vi "filter_active_tracks_for_mature_tracks.vi"(1 "All Active Tracks":T1[](array[typedef])) -> (0 "All Mature Tracks":T1[](array[typedef]))   [LabVIEW 2019]
uses:
  WormTrackCluster.ctl
  StimulusObject.lvclass
  TrackTerminationReasonEnum.ctl
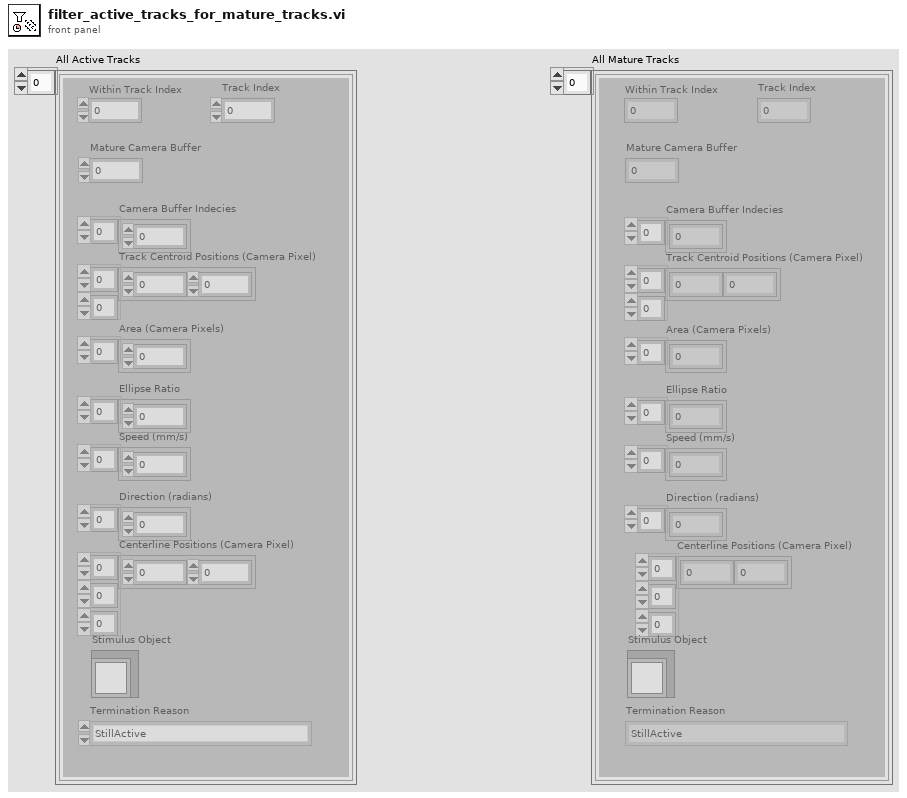
[diagram p1: front panel]
types:
  T1 = typedef "WormTrackCluster.ctl" = cluster{"Track Centroid Positions (Camera Pixel)":sgl[][], "Within Track Index":i32, "Camera Buffer Indecies":i32[], "Area (Camera Pixels)":i32[], "Speed (mm/s)":sgl[], "Direction (radians)":sgl[], "Centerline Positions (Camera Pixel)":sgl[][][], "Ellipse Ratio":sgl[], "Stimulus Object":refnum<class "StimulusObject.lvclass">, "Termination Reason":T2, "Track Index":i32, "Mature Camera Buffer":i32}
  T2 = typedef "TrackTerminationReasonEnum.ctl" = enum16{"StillActive", "MaxDisplacement", "NoBlobsLeft", "AreaIncrease", "AreaDecrease", "ExperimentEnded"}
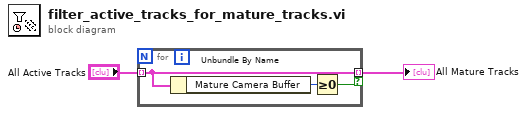
[diagram p0: block diagram]
diagram:
  n1 = for {
    tunnel: "All Active Tracks" -> [w5] mode=indexing
    tunnel: [w5] -> w1 mode=indexing if=w3
    n2 = Unbundle By Name(w5) -> ("Mature Camera Buffer"=w4:i32)
    n3 = Greater Or Equal To 0?(x=w4) -> (x >= 0?=w3:bool)
  }
  "All Mature Tracks" <- w1
